vi "Write Data.vi"(10 "Data":i32, 11 "HAL Interface Actor Task Msg in":refnum<class "HAL Interface Actor Task Msg.lvclass">) -> (3 "HAL Interface Actor Task Msg out":refnum<class "HAL Interface Actor Task Msg.lvclass">)   [LabVIEW 2024, in "HAL Interface Actor.lvlib" / "HAL Interface Actor Task Msg.lvclass"]
uses:
  HAL Interface Actor Task Msg.lvclass
  HAL Interface Actor Task Msg.lvclass/HAL Interface Actor Task Msg.ctl
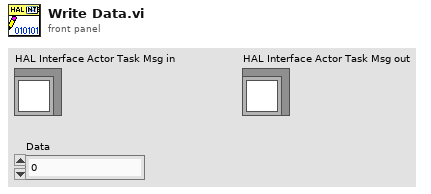
[diagram p1: front panel]
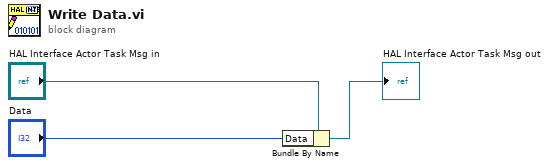
[diagram p0: block diagram]
diagram:
  n1 = Bundle By Name(cluster="HAL Interface Actor Task Msg in", "Data"="Data") -> (→"HAL Interface Actor Task Msg out":refnum<class "HAL Interface Actor Task Msg.lvclass">)
